vi "PH_VacuumControl.Config or Close.vi"(0 "i ref in":refnum<vi>, 2 "Action":u16(ring) items=["Configure", "Close"], 5 "error in (no error)":errorcluster) -> (14 "i ref out":refnum<vi>, 19 "error out":errorcluster)   [LabVIEW 2014, in "PH_VacuumControl.lvlib"]
doc: "This VI sets different essential things, writes GUI lements and own attributes, if \"Config\" is chosen, otherwise it closes the connection."
uses:
  PH_VacuumControl.lvlib
  PH_StatusHandler/PH_StatusHandler.Status.ctl
  instr.lib/AGCxxx/AGCxxx - Driver.lvlib
  PH_StatusHandler/PH_StatusHandler.lvlib
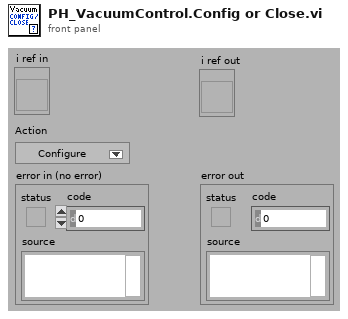
[diagram p1: front panel]
types:
  T1 = typedef "PH_StatusHandler.lvlib/PH_StatusHandler.Status.ctl" = i16
  T2 = typedef "PH_VacuumControl.lvlib/PH_VacuumControl.i attribute.ctl" = cluster{"GUI Refs":cluster{"Exit":refnum<vi>, "Set Unit":refnum<vi>, "Device found":refnum<vi>, "Busy":refnum<vi>, "State":refnum<vi>, "Delete":refnum<vi>, "Channels":refnum<vi>, "Channel Name":refnum<vi>, "Trend":refnum<vi>, "Logarithmic":refnum<vi>, "Limit reached":refnum<vi>, "Channel Name 1 MT":refnum<vi>, "Channel Name 2 MT":refnum<vi>, "Trend MT":refnum<vi>, "Logarithmic MT":refnum<vi>, "Limit reached MT":refnum<vi>}, "Device found":bool, "Busy":bool, "Selected Unit":i32, "Channels [mbar]":T3, "Channel Names":cluster{"Channel 1":string, "Channel 2":string, "Channel 3":string, "Channel 4":string, "Channel 5":string, "Channel 6":string}, "Status":T1, "AGCxxx VISA Cluster":T4, "Instr Firmware Revision":string, "Service IDs Pressure":cluster{"Channel 1":i32, "Channel 2":i32, "Channel 3":i32, "Channel 4":i32, "Channel 5":i32, "Channel 6":i32}, "Service IDs Limits":cluster{"Channel 1":i32, "Channel 2":i32, "Channel 3":i32, "Channel 4":i32, "Channel 5":i32, "Channel 6":i32}, "Trend":cluster{"Start Point":timestamp, "Pressures [mbar] Channel 1":dbl[], "Pressures [mbar] Channel 2":dbl[], "Pressures [mbar] Channel 3":dbl[], "Pressures [mbar] Channel 4":dbl[], "Pressures [mbar] Channel 5":dbl[], "Pressures [mbar] Channel 6":dbl[], "Timebase [s]":i32[], "Trend Channel":u16, "Start Fit":dbl, "Trend Channel 1 MT":u16, "Trend Channel 2 MT":u16, "Start or continue Fit MT":dbl, "Continue or start Fit MT":dbl, "Datasets strored":i32, "Dataarray Size":i32}, "Running":bool}
  T3 = typedef "PH_VacuumControl.lvlib/PH_VacuumControl.Channels.ctl" = cluster{"Channel 1":dbl, "Channel 2":dbl, "Channel 3":dbl, "Channel 4":dbl, "Channel 5":dbl, "Channel 6":dbl, "Name Channel 1":string, "Name Channel 2":string, "Name Channel 3":string, "Name Channel 4":string, "Name Channel 5":string, "Name Channel 6":string, "Upper Limit":dbl, "Upper Limit 2":dbl, "Upper Limit 3":dbl, "Upper Limit 4":dbl, "Upper Limit 5":dbl, "Upper Limit 6":dbl}
  T4 = typedef "AGCxxx - Driver.lvlib/AGCxxx VISA Control.ctl" = cluster{"VISA resource name":refnum<visa-resource-name>, "VISA Timeout Value (1000 ms)":u32, "Lock Timeout (1000 ms)":u32, "MAX Channel (6)":i32}
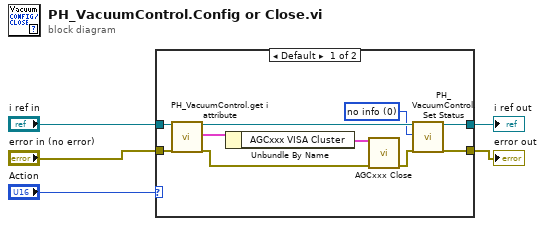
[diagram p0: block diagram]
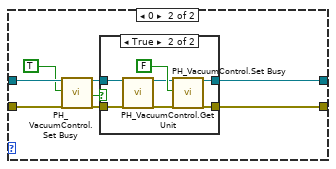
[diagram p2: hidden frame]
diagram:
  n1 = case shown="Default" "Action" {
    tunnel: [w7 w23] -> w5
    tunnel: "error in (no error)" -> [w14 w22]
    tunnel: [w9 w21] -> w3
    tunnel: "i ref in" -> [w15 w20]
    frame Default {
      w6 = T1 0 items=["no info", "off/false/out", "on/true/in", "Failure", "Alarm", "Status 1", "Status 2", "Status 3"] ("State")
      n2 = call "PH_VacuumControl.get i attribute.vi"("i ref in"=w15, "error in (no error)"=w14) -> ("i ref out"=w10:refnum<vi>, "i attribute"=w13:T2, "error out"=w11:errorcluster)  [unwired: 15 in]
      n3 = Unbundle By Name(w13) -> ("AGCxxx VISA Cluster"=w12:T4)
      n4 = call "AGCxxx Close.vi"("AGCxxx VISA Cluster"=w12, "error in (no error)"=w11) -> ("error out"=w8:errorcluster)  [unwired: 13 in]
      n5 = call "PH_VacuumControl.Set Status.vi"("i ref in"=w10, "Status"=w6, "error in (no error)"=w8) -> ("i ref out"=w9:refnum<vi>, "error out"=w7:errorcluster)  [unwired: 15 in]
    }
    frame 0 {
      n6 = call "PH_VacuumControl.Set Busy.vi"("i ref in"=w20, "Busy"=TRUE, "error in (no error)"=w22) -> ("i ref out"=w17:refnum<vi>, "changed"=w16:bool, "error out"=w18:errorcluster)  [unwired: 14 in]
      n7 = case shown="True" w16 {
        tunnel: [w24 w31] -> w23
        tunnel: [w25 w30] -> w21
        tunnel: w18 -> [w24 w29]
        tunnel: w17 -> [w25 w28]
        frame False {
        }
        frame True {
          n8 = call "PH_VacuumControl.Get Unit.vi"("i ref in"=w28, "error in (no error)"=w29) -> ("i ref out"=w27:refnum<vi>, "error out"=w26:errorcluster)  [unwired: 16 in]
          n9 = call "PH_VacuumControl.Set Busy.vi"("i ref in"=w27, "Busy"=FALSE, "error in (no error)"=w26) -> ("i ref out"=w30:refnum<vi>, "error out"=w31:errorcluster)  [unwired: 14 in, 1 out]
        }
      }
    }
  }
  "error out" <- w5
  "i ref out" <- w3
